vi "configuration.get.vi"(8 "error in":errorcluster) -> (0 "error out":errorcluster, 3 "configuration":T1={"Position"=enum."Left", "Note Length"=50.0} {"Note Length" format="%#_13g"})   [LabVIEW 2020]
uses:
  configuration.ctl
  <vilib>/Utility/config.llb/NI_LVConfig.lvlib
  <userlib>/_OpenG.lib/variantconfig/variantconfig.llb/openg_variant_configuration_file.lvlib
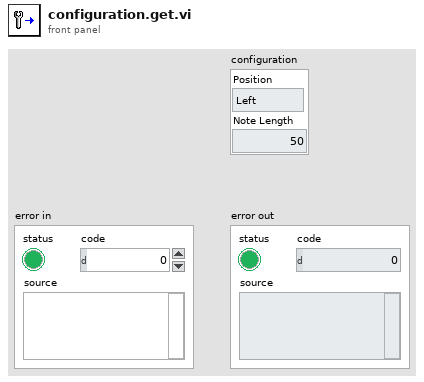
[diagram p1: front panel]
types:
  T1 = typedef "configuration.ctl" = cluster{"Position":enum16{"Top", "Left", "Botom", "Right"}, "Note Length":dbl}
  T2 = typedef "NI_LVConfig.lvlib/Config Data RefNum.ctl" = refnum<k1>
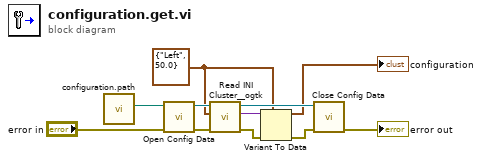
[diagram p0: block diagram]
diagram:
  w8 = T1 {"Position"=enum."Left", "Note Length"=50.0} ("configuration")
  n1 = call "configuration.path.vi"() -> ("configuration file"=w1:path)  [unwired: 11 in]
  n2 = call <vilib>:"Open Config Data.vi"("error in (no error)"="error in", "configuration file path"=w1) -> ("error out"=w10:errorcluster, "refnum"=w11:T2)  [unwired: 7 in, 1 out]
  n3 = call <userlib>:"Read INI Cluster__ogtk.vi"("error in (no error)"=w10, "INI Fomatted Cluster Type"=w8, "refnum"=w11) -> ("error out"=w5:errorcluster, "INI Fomatted Cluster"=w7:variant, "dup refnum"=w9:T2)  [unwired: 4 in, 2 out]
  n4 = Variant To Data(error in=w5, type=w8, Variant=w7) -> (data=→"configuration":T1, error out=w4:errorcluster)
  n5 = call <vilib>:"Close Config Data.vi"("error in (no error)"=w4, "refnum"=w9) -> ("error out"=→"error out":errorcluster)  [unwired: 8 in, 1 out]
